vi "Datos del Vehiculo.vi"(7 "#Pasajeros":u16, 8 "error in (no error)":errorcluster, 9 "Tipo Motor":enum16{"Eléctrico", "Gasolina"}(ring), 10 "Ambiente de operacion":enum16{"Acuático", "Terrestre", "Aereo"}(ring), 11 "Vehiculo de Motor in":refnum<class "Vehiculo de Motor.lvclass">) -> (0 "error out":errorcluster, 3 "Vehiculo de Motor out":refnum<class "Vehiculo de Motor.lvclass">)   [LabVIEW 2020, in "Vehiculo de Motor.lvclass"]
uses:
  Vehiculo de Motor.lvclass
  Vehiculo de Motor.lvclass/Vehiculo de Motor.ctl
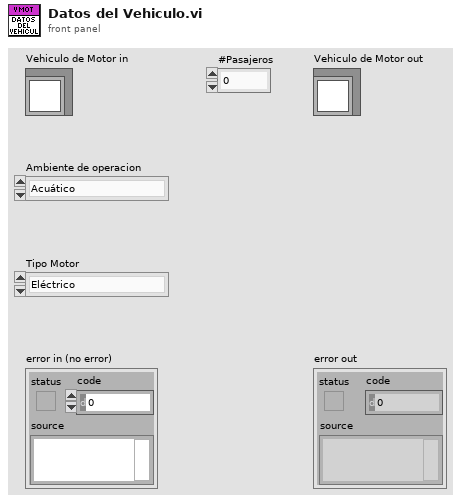
[diagram p1: front panel]
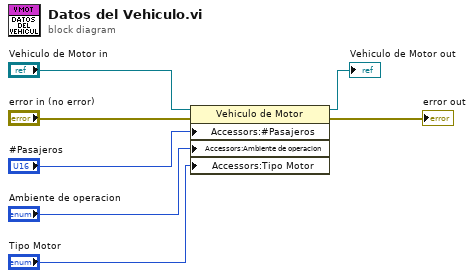
[diagram p0: block diagram]
diagram:
  n1 = property class="Vehiculo de Motor"(reference="Vehiculo de Motor in", error in="error in (no error)", "Accessors:#Pasajeros"="#Pasajeros", "Accessors:Ambiente de operacion"="Ambiente de operacion", "Accessors:Tipo Motor"="Tipo Motor") -> (reference out=→"Vehiculo de Motor out":refnum<class "Vehiculo de Motor.lvclass">, error out=→"error out":errorcluster)
